vi "衬丝头检测结果数据库判定.vi"(8 "error in (no error)":errorcluster caption="错误输入（无错误）", 10 "衬丝头检测结果":bool, 11 "ADODB._Connection In":refnum<k7>) -> (0 "error out":errorcluster caption="错误输出", 3 "ADODB._Connection Out":refnum<k7>)   [LabVIEW 2017]
panel:
  out "连接的字符串 4":string
  out "连接的字符串":string
  out "Data":string[][](array[string])
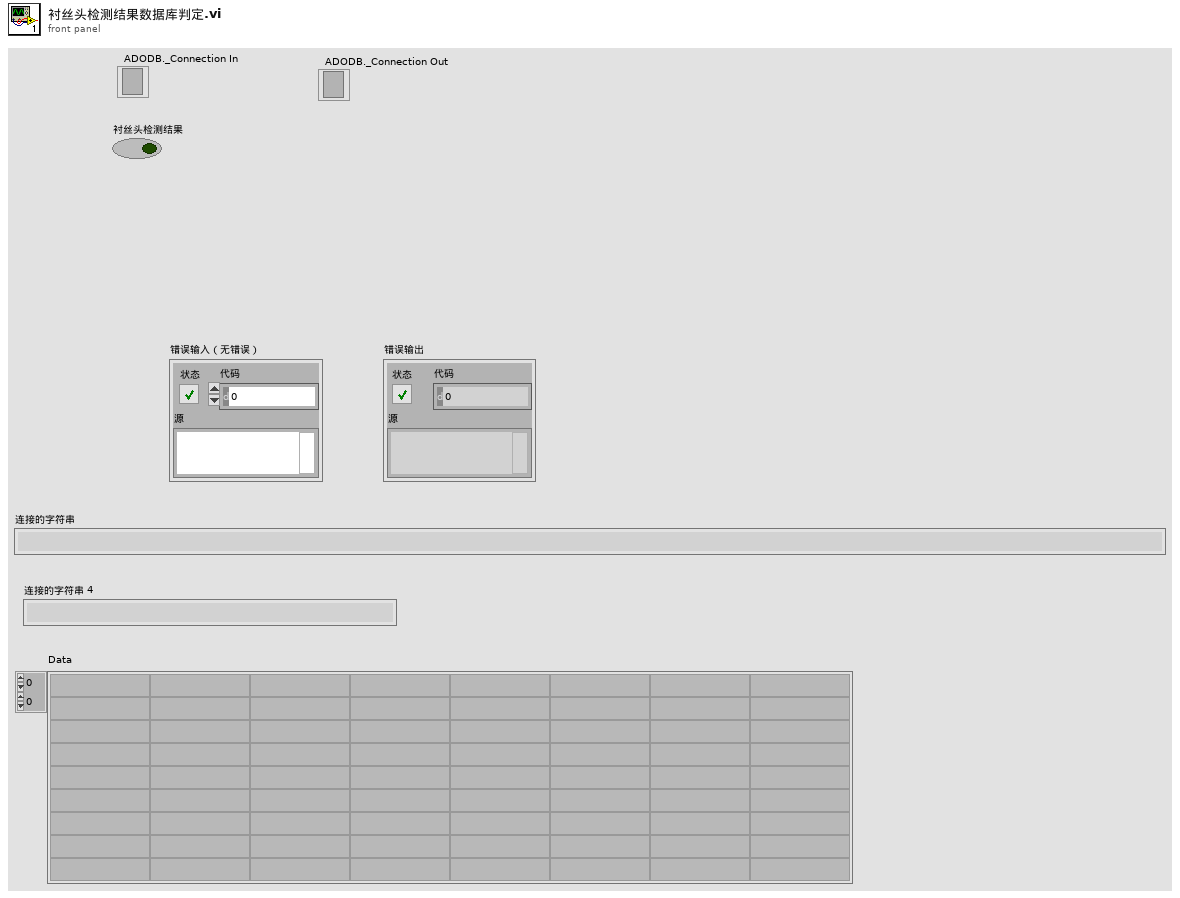
[diagram p1: front panel]
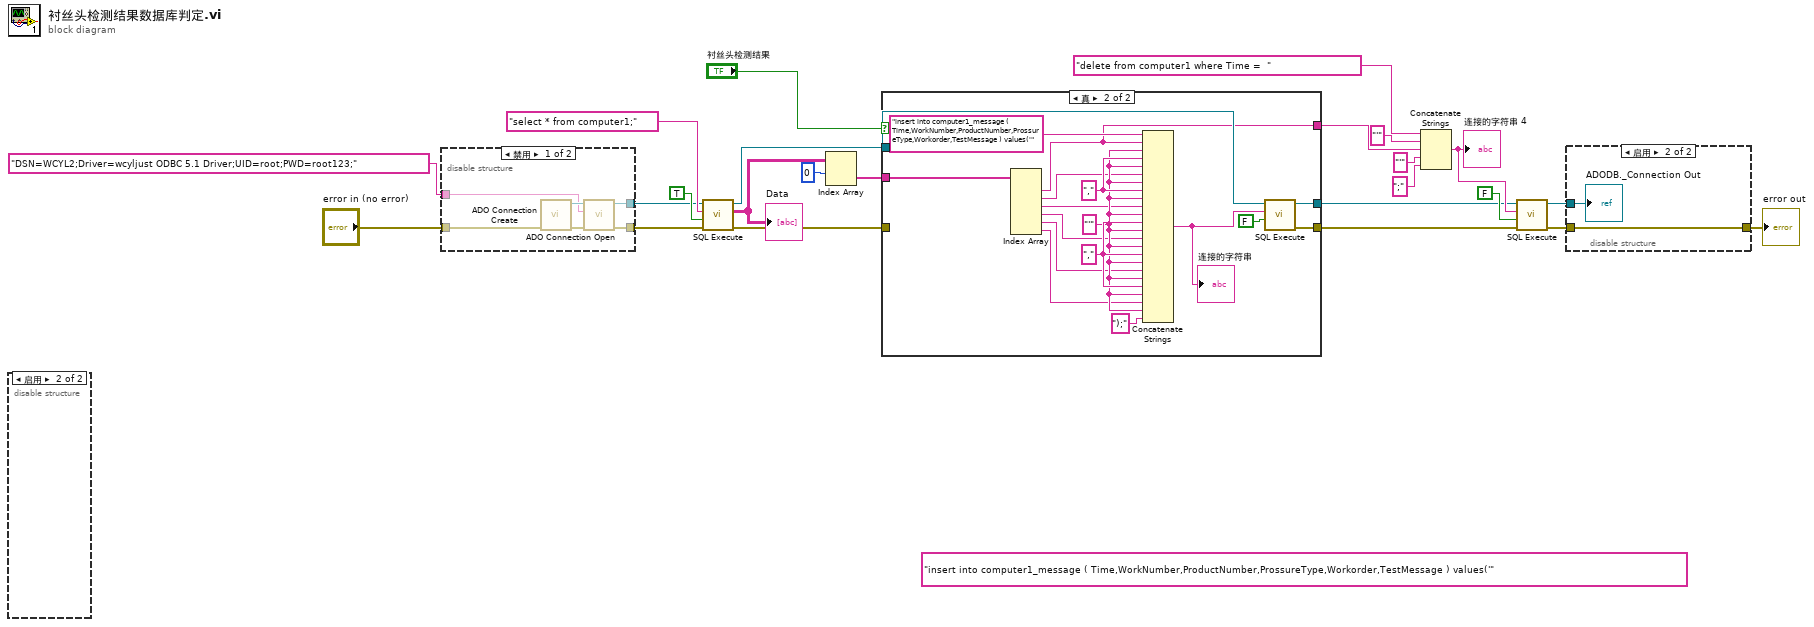
[diagram p0: block diagram]
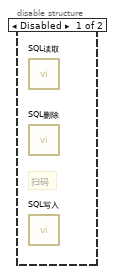
[diagram p2: hidden frame]
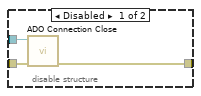
[diagram p3: hidden frame]
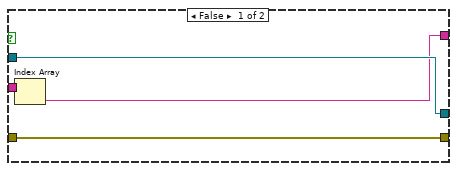
[diagram p4: hidden frame]
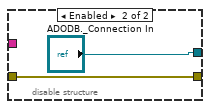
[diagram p5: hidden frame]
diagram:
  (unwired) "insert into computer1_message ( Time,WorkNumber,ProductNumber,ProssureType,Workorder,TestMessage ) values('" ("Command Text")
  n1 = disable-structure shown="启用" {
    frame Disabled {
      # "扫码"
      n2 = call "SQL读取.vi"() -> ()  [unwired: 6 in, 6 out]
      n3 = call "SQL删除.vi"() -> ()  [unwired: 15 in, 1 out]
      n4 = call "SQL写入.vi"() -> ()  [unwired: 18 in, 2 out]
    }
    frame Enabled {
    }
  }
  n5 = disable-structure shown="禁用" {
    disable-tunnel: "DSN=WCYL2;Driver=wcyljust ODBC 5.1 Driver;UID=root;PWD=root123;" ("ConnectionString") -> [w28 _]
    disable-tunnel: [w27 "ADODB._Connection In"] -> w20
    disable-tunnel: [w26 w32] -> w19
    disable-tunnel: "error in (no error)" -> [w25 w32]
    frame Disabled {
      n6 = call <userlib>:"ADO Connection Create.vi"("error in (no error)"=w25) -> ("error out"=w29:errorcluster, "ADODB._Connection Out"=w30:refnum<k7>)  [unwired: 9 in]
      n7 = call <userlib>:"ADO Connection Open.vi"("error in (no error)"=w29, "ConnectionString"=w28, "ADODB._Connection In"=w30) -> ("error out"=w26:errorcluster, "ADODB._Connection Out"=w27:refnum<k7>)  [unwired: 7 in]
    }
    frame Enabled {
    }
  }
  n8 = call <userlib>:"SQL Execute.vi"("error in (no error)"=w19, "Return Data (T)"=TRUE, "Command Text"="select * from computer1;", "ADODB._Connection In"=w20) -> ("error out"=w15:errorcluster, "Data"=w1:string[][], "ADODB._Connection Out"=w16:refnum<k7>)  [unwired: 4 in, 1 out]
  "Data" <- w1
  n9 = Index Array(array=w1, index (row)=0 ("索引 (行)")) -> (element=w3:string[])  [unwired: 1 in]
  n10 = case shown="真" "衬丝头检测结果" {
    tunnel: w16 -> [w35 w52]
    tunnel: w15 -> [w36 _]
    tunnel: [w35 w51] -> w7
    tunnel: [w36 w50] -> w5
    tunnel: w3 -> [w34 w43]
    tunnel: [w33 w42] -> w2
    frame False {
      n11 = Index Array(array=w34) -> (element=w33:string)  [unwired: 1 in]
    }
    frame True {
      w46 = "'" ("字符串")
      w47 = "," ("字符串")
      w49 = "," ("字符串")
      n12 = Index Array(array=w43) -> (element #1=w42:string, element #2=w41:string, element #3=w40:string, element #4=w39:string, element #5=w38:string, element #6=w37:string)  [unwired: 6 in]
      n13 = Concatenate Strings("insert into computer1_message ( Time,WorkNumber,ProductNumber,ProssureType,Workorder,TestMessage ) values('" ("Command Text"), w42, w46, w49, w46, w41, w46, w49, w46, w40, w46, w47, w46, w39, w46, w47, w46, w38, w46, w47, w46, w37, w46, ");" ("字符串")) -> (w44:string)
      "连接的字符串" <- w44
      n14 = call <userlib>:"SQL Execute.vi"("Return Data (T)"=FALSE, "Command Text"=w44, "ADODB._Connection In"=w52) -> ("error out"=w50:errorcluster, "ADODB._Connection Out"=w51:refnum<k7>)  [unwired: 5 in, 2 out]
    }
  }
  n15 = Concatenate Strings("delete from computer1 where Time =  " ("Command Text"), "'" ("字符串"), w2, "'" ("字符串"), ";" ("字符串")) -> (w9:string)
  "连接的字符串 4" <- w9
  n16 = call <userlib>:"SQL Execute.vi"("error in (no error)"=w5, "Return Data (T)"=FALSE, "Command Text"=w9, "ADODB._Connection In"=w7) -> ("error out"=w4:errorcluster, "ADODB._Connection Out"=w6:refnum<k7>)  [unwired: 4 in, 2 out]
  n17 = disable-structure shown="启用" {
    disable-tunnel: [w56 w58] -> w14
    disable-tunnel: w6 -> [w55 w57]
    disable-tunnel: w4 -> [w54 w58]
    frame Disabled {
      n18 = call <userlib>:"ADO Connection Close.vi"("error in (no error)"=w54, "ADODB._Connection In"=w55) -> ("error out"=w56:errorcluster)  [unwired: 8 in, 1 out]
    }
    frame Enabled {
      "ADODB._Connection Out" <- w57
    }
  }
  "error out" <- w14
